vi "To Bool Tree Data.vi"(10 "Boolean":bool) -> (3 "Bool Tree Data":refnum<class "Bool.lvclass">)   [LabVIEW 2016, in "Bool.lvclass"]
uses:
  Bool.lvclass
  Bool.lvclass/Bool.ctl
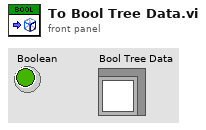
[diagram p1: front panel]
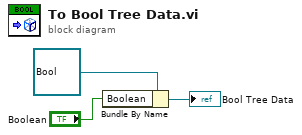
[diagram p0: block diagram]
diagram:
  n1 = Bundle By Name(cluster=refnum<class "Bool.lvclass"> refnum ("Bool in"), "Boolean"="Boolean") -> (→"Bool Tree Data":refnum<class "Bool.lvclass">)
